vi "ModifyChnlHW.vi"(8 "error in (no error)":errorcluster, 11 "BME_DG_G05P2_Chnl in":refnum<class "BME_DG_G05P2_Chnl.lvclass">) -> (0 "error out":errorcluster, 3 "BME_DG_G05P2_Chnl out":refnum<class "BME_DG_G05P2_Chnl.lvclass">)   [LabVIEW 2009, in "POLARIS BME DG.lvlib" / "BME_DG_G05P2_Chnl.lvclass"]
uses:
  BME_DG_G05P2_Chnl.lvclass
  BME_DG_G05P2_Chnl.lvclass/BME_DG_G05P2_Chnl.ctl
  POLARIS BME DG.lvlib
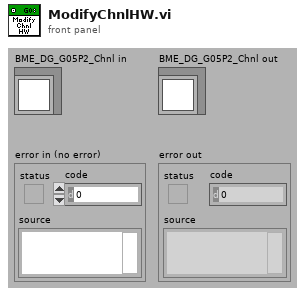
[diagram p1: front panel]
types:
  T1 = typedef "POLARIS BME DG.lvlib/ChnlSettings.ctl" = cluster{" Delay (µs)":dbl, "On?":bool, "PositiveVoltage?":bool, "50OhmTerminated? ":bool, "25OhmOutput?":bool}
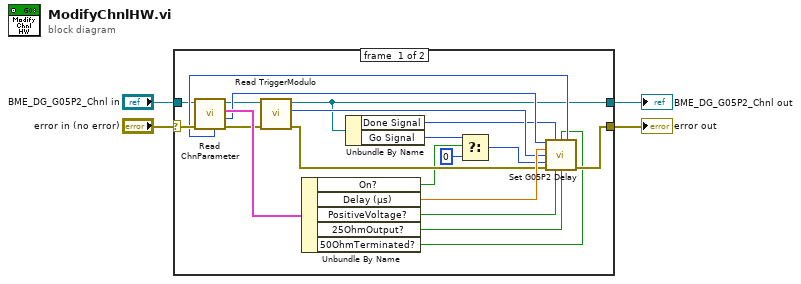
[diagram p0: block diagram]
diagram:
  n1 = case shown="No Error" "error in (no error)" {
    selector: "error in (no error)" -> [w23 w26]
    tunnel: [w22 w26] -> w1
    tunnel: [w11 w25] -> w3
    tunnel: "BME_DG_G05P2_Chnl in" -> [w16 w25]
    frame #0 {
      n2 = call-dynamic "Read ChnParameter.vi"("error in (no error)"=w23, "BME_DG_Chnl in"=w16) -> ("error out"=w15:errorcluster, "Nr"=w20:i32, "ChnParemater"=w24:T1, "BME_DG_Chnl out"=w12:refnum<class "BME_DG_G05P2_Chnl.lvclass">, "DG Nr"=w19:i32)  [unwired: 4 in, 1 out]
      n3 = call-dynamic "Read TriggerModulo.vi"("error in (no error)"=w15, "BME_DG_G05_Chnl in"=w12) -> ("error out"=w14:errorcluster, "TriggerModulo"=w13:i32, "BME_DG_G05_Chnl out"=w11:refnum<class "BME_DG_G05P2_Chnl.lvclass">)  [unwired: 7 in]
      n4 = Unbundle By Name(w24) -> ("On?"=w7:bool, "Delay (µs)"=w21:dbl, "PositiveVoltage?"=w18:bool, "25OhmOutput?"=w17:bool, "50OhmTerminated?"=w9:bool)
      n5 = Unbundle By Name(w11) -> ("Done Signal"=w10:u32, "Go Signal"=w6:u32)
      n6 = Select(t=w6, s=w7, f=u32 0) -> (s? t:f=w5:u32)
      n7 = call "Set G05P2 Delay.vi"("Channel"=w20, "DoneSignal"=w10, "Terminate"=w9, "DG Number"=w19, "Delay (µs)"=w21, "OutputModulo"=w13, "GoSignal"=w5, "error in (no error)"=w14, "Polarity"=w18, "High Drive"=w17) -> ("error out"=w22:errorcluster)  [unwired: 5 in]
    }
    frame #1 {
    }
  }
  "error out" <- w1
  "BME_DG_G05P2_Chnl out" <- w3
